vi "ADI_IMU_ADIS16470_WriteRegister.vi"(8 "error in (no error)":errorcluster, 9 "Data":u16=2049, 10 "Register":T1=54 items=["SMPL_PRD"=54, "SENS_AVG"=56, "MSC_CTRL"=52, "ERROR_FLAGS"=60, "TEMP"=44, "BARO"=40, "Z_MAG"=36, "Y_MAG"=32, "X_MAG"=28, "Z_ACCEL"=24, "Y_ACCEL"=20, "X_ACCEL"=16, "Z_GYRO"=12, "Y_GYRO"=8, "X_GYRO"=4, "PID"=86], 11 "SPIDevRef in":T2) -> (0 "error out":errorcluster, 3 "SPIDevRef out":T2)   [LabVIEW 2018, in "ADIS16470_IMU.lvlib"]
uses:
  ADIS16470_IMU.lvlib
  <vilib>/Rock Robotics/WPI/SPI/WPI_SPIDevRef.ctl
  <vilib>/Rock Robotics/SystemInterfaces/spilib/spi_bus.ctl
  ADI_IMU_ADIS16470_Registers.ctl
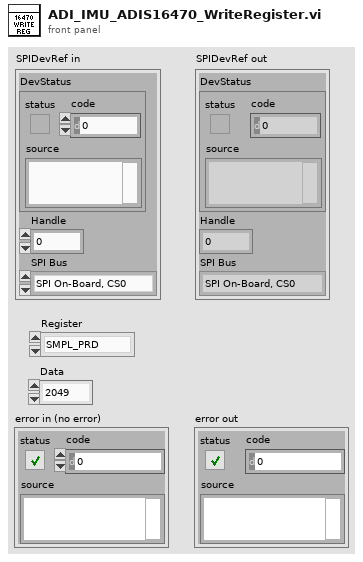
[diagram p1: front panel]
types:
  T1 = typedef "ADIS16470_IMU.lvlib/ADI_IMU_ADIS16470_Registers.ctl" = u8
  T2 = typedef "WPI_SPIDevRef.ctl" = cluster{"DevStatus":errorcluster, "Handle":i32, "SPI Bus":T3}
  T3 = typedef "spi_bus.ctl" = enum16{"SPI On-Board, CS0", "SPI On-Board, CS1", "SPI On-Board, CS2", "SPI On-Board, CS3", "SPI MXP", "Invalid"}
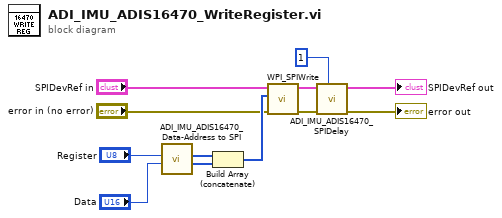
[diagram p0: block diagram]
diagram:
  n1 = call "ADI_IMU_ADIS16470_Data-Address to SPI.vi"("Data"="Data", "Address"="Register") -> ("High Word"=w1:u8[], "Low Word"=w2:u8[])  [unwired: 8 in]
  n2 = Build Array (concatenate)(w2, w1) -> (w12:u8[])
  n3 = call <vilib>:"WPI_SPIWrite.vi"("error in (no error)"="error in (no error)", "Data To Send"=w12, "SPIDevRef"="SPIDevRef in") -> ("error out"=w3:errorcluster, "SPIDevRef"=w7:T2)  [unwired: 7 out]
  n4 = call "ADI_IMU_ADIS16470_SPIDelay.vi"("Wait (ms)"=u32 1, "error in"=w3, "SPIDevRef in"=w7) -> ("error out"=→"error out":errorcluster, "SPIDevRef out"=→"SPIDevRef out":T2)  [unwired: 7 in]
